vi "Get Style.vi"(8 "error in (no error)":errorcluster, 11 "xwpfRun in":refnum<class "xwpfRun.lvclass">) -> (0 "error out":errorcluster, 2 "Styles.lvlib:Style.lvclass":refnum<class "Style.lvclass">, 3 "xwpfRun out":refnum<class "xwpfRun.lvclass">)   [LabVIEW 2017, in "Word_Specific.lvlib" / "xwpfRun.lvclass"]
uses:
  xwpfRun.lvclass
  Styles/Style/Style.lvclass
  xwpfRun.lvclass/xwpfRun.ctl
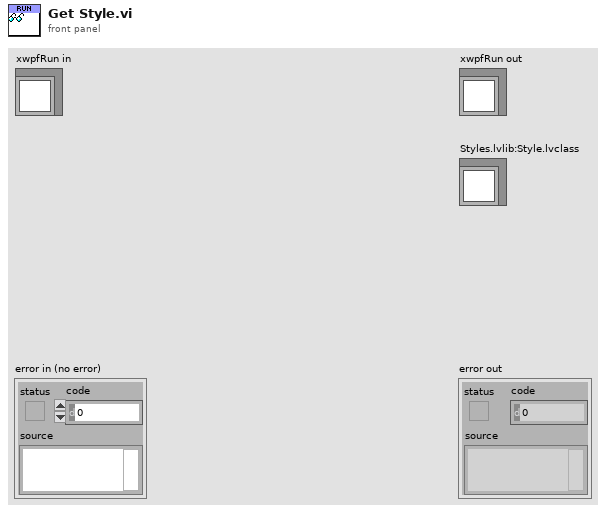
[diagram p1: front panel]
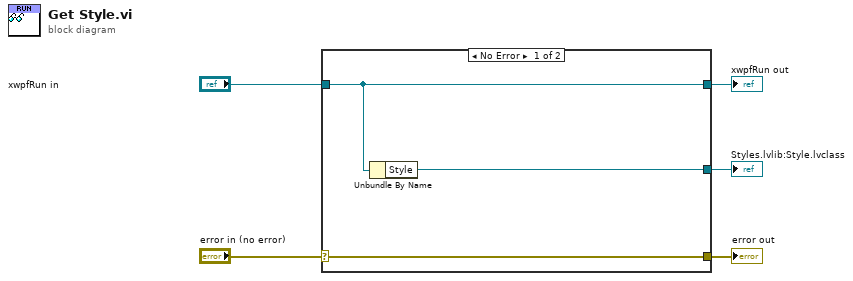
[diagram p0: block diagram]
diagram:
  n1 = case shown="No Error" "error in (no error)" {
    selector: "error in (no error)" -> [w8 w9]
    tunnel: [w8 w9] -> w4
    tunnel: [w7 w10] -> w2
    tunnel: "xwpfRun in" -> [w7 w10]
    tunnel: [w6 _] -> w1
    frame No Error {
      n2 = Unbundle By Name(w7) -> ("Style"=w6:refnum<class "Style.lvclass">)
    }
    frame Error {
    }
  }
  "error out" <- w4
  "xwpfRun out" <- w2
  "Styles.lvlib:Style.lvclass" <- w1
